vi "LabVIEW controller.vi"() -> ()   [LabVIEW 2013]
uses:
  <vilib>/NXT/NXT Controls/ConnectionType.ctl
  <vilib>/NXT/Subs/MotorOutput.ctl
  <vilib>/NXT/NXTIO Xnodes/NXTIONodeSubVIs/LEGOStopAllMotors.vi
  <vilib>/NXT/NXTIO Xnodes/NXTIOXNode/NXTIO.xnode
  <vilib>/NXT/Subs/LVHSConnector.ctl
  <vilib>/NXT/LegoClasses/BrickReference/BrickReference.lvclass
panel:
  out "Y":dbl
  out "X":dbl
  in  "YFile":path
  in  "XFile":path
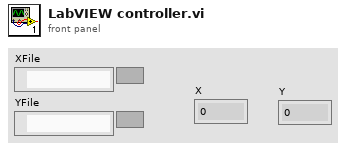
[diagram p1: front panel]
types:
  T1 = typedef "MotorOutput.ctl" = u8
  T2 = typedef "ConnectionType.ctl" = enum16{"Bluetooth", "USB", "WiFi"}
  T3 = typedef "LVHSConnector.ctl" = refnum<class "BrickReference.lvclass">
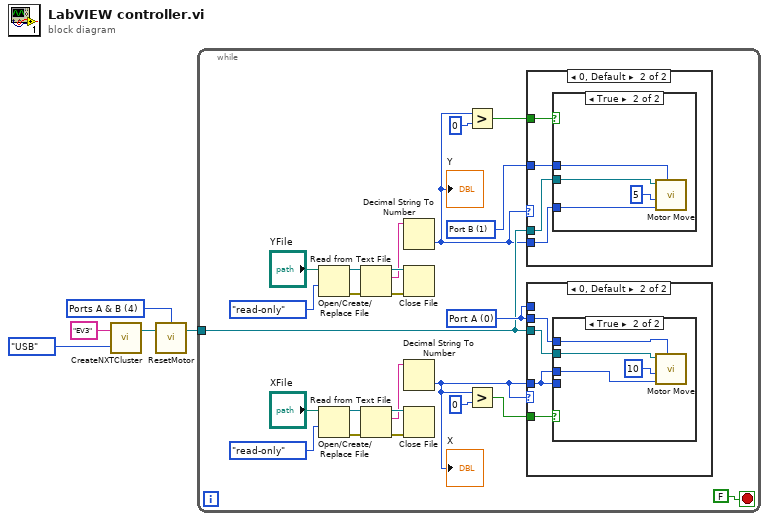
[diagram p0: block diagram]
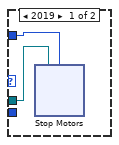
[diagram p2: hidden frame]
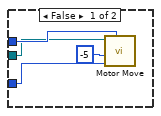
[diagram p3: hidden frame]
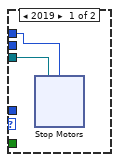
[diagram p4: hidden frame]
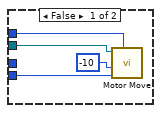
[diagram p5: hidden frame]
diagram:
  w2 = T1 4 items=["Port A"=0, "Port B"=1, "Port C"=2, "Ports A & B"=4, "Ports A & C"=5, "Ports B & C"=6, "All Ports"=3] ("Port (All Ports)")
  n1 = call <vilib>:"CreateNXTCluster.vi"("Connection Type"=ConnectionType."USB", "NXT/EV3 name"="EV3") -> ("NXT/EV3"=w3:T3)  [unwired: 2 in]
  n2 = call <vilib>:"ResetMotor.vi"("NXT/EV3"=w3, "Port (All Ports)"=w2) -> ("NXT/EV3"=w1:T3)  [unwired: 2 in]
  n3 = while {
    tunnel: w1 -> [w12]
    stop <- FALSE stop-if-true
    w13 = T1 1 items=["Port A"=0, "Port B"=1, "Port C"=2, "Ports A & B"=4, "Ports A & C"=5, "Ports B & C"=6, "All Ports"=3] ("Output Port (All Ports)")
    w14 = T1 0 items=["Port A"=0, "Port B"=1, "Port C"=2, "Ports A & B"=4, "Ports A & C"=5, "Ports B & C"=6, "All Ports"=3] ("Output Port (All Ports)")
    n4 = Open/Create/Replace File(file path (use dialog)="YFile", access (0:read/write)=enum16{"read/write", "read-only", "write-only"}."read-only") -> (refnum out=w27:refnum<file>, error out=w26:errorcluster)  [unwired: 4 in, 1 out]
    n5 = Open/Create/Replace File(file path (use dialog)="XFile", access (0:read/write)=enum16{"read/write", "read-only", "write-only"}."read-only") -> (refnum out=w22:refnum<file>, error out=w21:errorcluster)  [unwired: 4 in, 1 out]
    n6 = Read from Text File(file (use dialog)=w27, error in=w26) -> (refnum out=w25:refnum<file>, text=w18:string, error out=w24:errorcluster)  [unwired: 2 in, 1 out]
    n7 = Read from Text File(file (use dialog)=w22, error in=w21) -> (refnum out=w20:refnum<file>, text=w17:string, error out=w19:errorcluster)  [unwired: 2 in, 1 out]
    n8 = Decimal String To Number(string=w18) -> (number=w7:i32)  [unwired: 2 in, 1 out]
    "Y" <- w7
    n9 = Close File(refnum=w25, error in=w24) -> ()  [unwired: 2 out]
    n10 = Decimal String To Number(string=w17) -> (number=w10:i32)  [unwired: 2 in, 1 out]
    "X" <- w10
    n11 = Close File(refnum=w20, error in=w19) -> ()  [unwired: 2 out]
    n12 = Greater?(x=w7, y=0) -> (0:w8:bool)
    n13 = Greater?(x=w10, y=0) -> (0:w11:bool)
    n14 = case shown="0, Default" w7 {
      tunnel: w13 -> [w31 w40]
      tunnel: w7 -> [_ w39]
      tunnel: w12 -> [w30 w38]
      tunnel: w8 -> [_ w37]
      frame 2019 {
        n15 = xnode "Stop Motors"("Motors"=w31, "NXT/EV3"=w30) -> ()  [unwired: 1 out]
      }
      frame 0, Default {
        n16 = case shown="True" w37 {
          tunnel: w40 -> [w43 w48]
          tunnel: w39 -> [w41 w46]
          tunnel: w38 -> [w42 w45]
          frame False {
            n17 = call "Motor Move.vi"("Output Port (All Ports)"=w43, "Angle of Rotation (360)"=w41, "Power (75)"=-5, "NXT/EV3 2"=w42) -> ()  [unwired: 7 in, 1 out]
          }
          frame True {
            n18 = call "Motor Move.vi"("Output Port (All Ports)"=w48, "Angle of Rotation (360)"=w46, "Power (75)"=5, "NXT/EV3 2"=w45) -> ()  [unwired: 7 in, 1 out]
          }
        }
      }
    }
    n19 = case shown="0, Default" w10 {
      tunnel: w11 -> [_ w59]
      tunnel: w12 -> [w49 w58]
      tunnel: w14 -> [_ w57]
      tunnel: w10 -> [_ w56]
      tunnel: w14 -> [w50 _]
      frame 2019 {
        n20 = xnode "Stop Motors"("Motors"=w50, "NXT/EV3"=w49) -> ()  [unwired: 1 out]
      }
      frame 0, Default {
        n21 = case shown="True" w59 {
          tunnel: w58 -> [w61 w67]
          tunnel: w57 -> [w62 w66]
          tunnel: w56 -> [w60 _]
          tunnel: w56 -> [_ w64]
          frame False {
            n22 = call "Motor Move.vi"("Output Port (All Ports)"=w62, "Angle of Rotation (360)"=w60, "Power (75)"=-10, "NXT/EV3 2"=w61) -> ()  [unwired: 7 in, 1 out]
          }
          frame True {
            n23 = call "Motor Move.vi"("Output Port (All Ports)"=w66, "Angle of Rotation (360)"=w64, "Power (75)"=10, "NXT/EV3 2"=w67) -> ()  [unwired: 7 in, 1 out]
          }
        }
      }
    }
  }
